vi "Get V50s (SubVI).vi"(0 "recordset data":string[][](array[string])) -> (1 "V50 Array":dbl[](array[numeric]), 2 "V50 Table":string[][](array[string]), 3 "lastVelocity":dbl)   [LabVIEW 2010]
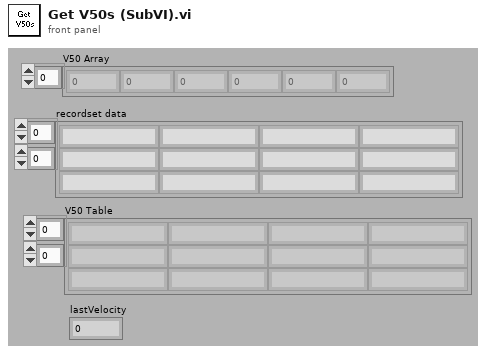
[diagram p1: front panel]
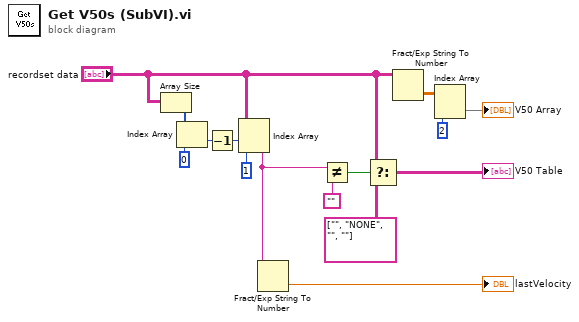
[diagram p0: block diagram]
diagram:
  n1 = Array Size(array="recordset data") -> (size(s)=w7:i32[])
  n2 = Index Array(array=w7, index=0 ("Index")) -> (element=w5:i32)
  n3 = Decrement(x=w5) -> (x-1=w4:i32)
  n4 = Index Array(array="recordset data", index (row)=w4, index (col)=1 ("Disabled Index (col)")) -> (element=w3:string)
  n5 = Fract/Exp String To Number(string=w3) -> (number=→"lastVelocity":dbl)  [unwired: 1 in, 3 out]
  n6 = Not Equal?(x=w3, y="" ("Empty String Constant")) -> (x != y?=w8:bool)
  n7 = Select(t="recordset data", s=w8, f=string[][] [["", "NONE"], ["", ""]]) -> (s? t:f=→"V50 Table":string[][])
  n8 = Fract/Exp String To Number(string="recordset data") -> (number=w13:dbl[][])  [unwired: 1 in, 3 out]
  n9 = Index Array(array=w13, index (col)=2 ("Disabled Index (col)")) -> (element=→"V50 Array":dbl[])  [unwired: 1 in]
